vi "CalculateBestY.vi"(8 "error in (no error)":errorcluster, 9 "Point":dbl[](array[numeric]), 10 "Game":refnum<class "Game.lvclass">, 11 "Evaluator in":refnum<class "Evaluator.lvclass">) -> (0 "error out":errorcluster, 2 "Game out":refnum<class "Game.lvclass">, 3 "Evaluator out":refnum<class "Evaluator.lvclass">)   [LabVIEW 2023, in "Evaluator.lvclass"]
uses:
  Evaluator.lvclass
  Game_class/Game.lvclass
  Evaluator.lvclass/Evaluator.ctl
  Game_class/Game.lvclass/Game.ctl
  Game_class/Read Utilities.lvclass.vi
  Game_class/Write Utilities.lvclass.vi
  Utilities_class/Utilities.lvclass
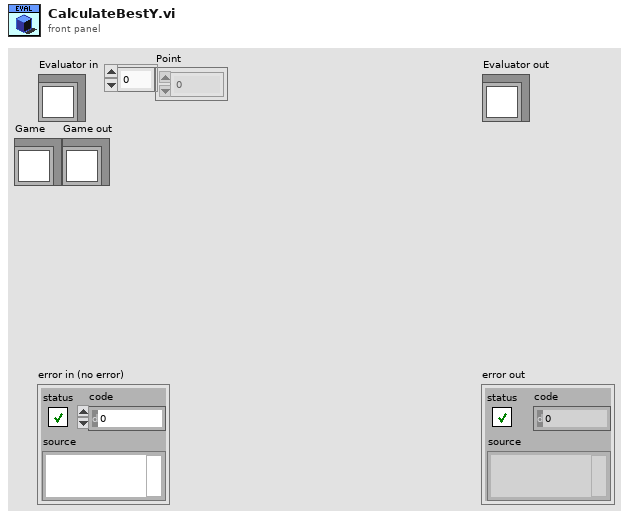
[diagram p1: front panel]
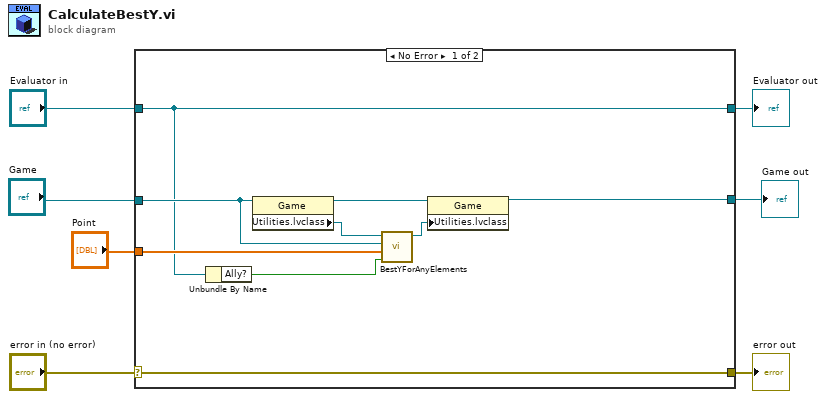
[diagram p0: block diagram]
diagram:
  n1 = case shown="No Error" "error in (no error)" {
    selector: "error in (no error)" -> [w16 w19]
    tunnel: [w16 w19] -> w6
    tunnel: [w9 w18] -> w4
    tunnel: "Evaluator in" -> [w9 w18]
    tunnel: "Game" -> [w12 w17]
    tunnel: [w11 w17] -> w2
    tunnel: "Point" -> [w10 _]
    frame No Error {
      n2 = Unbundle By Name(w9) -> ("Ally?"=w8:bool)
      n3 = property class="Game"(reference=w12) -> (reference out=w13:refnum<class "Game.lvclass">, "Utilities.lvclass"=w15:refnum<class "Utilities.lvclass">)  [unwired: 1 in, 1 out]
      n4 = call "BestYForAnyElements.vi"("inimigos"=w8, "Position to be analyzed"=w10, "Game"=w12, "Utilities in"=w15) -> ("Utilities out"=w14:refnum<class "Utilities.lvclass">)  [unwired: 4 in, 3 out]
      n5 = property class="Game"(reference=w13, "Utilities.lvclass"=w14) -> (reference out=w11:refnum<class "Game.lvclass">)  [unwired: 1 in, 1 out]
    }
    frame Error {
    }
  }
  "error out" <- w6
  "Evaluator out" <- w4
  "Game out" <- w2
